vi "To Variant.vi"(0 "Base in":refnum<class "KDemoBase.lvclass">, 11 "error in (no error)":errorcluster) -> (4 "Base out":refnum<class "KDemoBase.lvclass">, 8 "Array":variant[](array[variant]), 15 "error out":errorcluster)   [LabVIEW 2015, in "KDemoBase.lvclass"]
uses:
  KDemoBase.lvclass
  KDemoBase.lvclass/KDemoBase.ctl
  KObject Class/KObject.lvclass
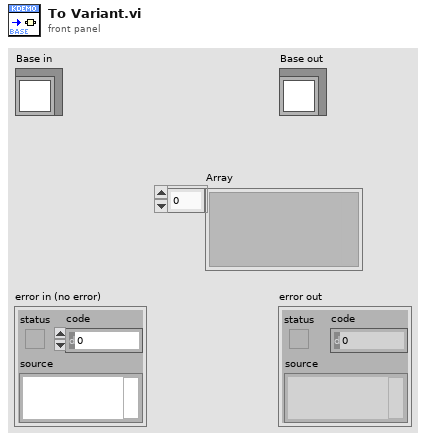
[diagram p1: front panel]
types:
  T1 = typedef "KDemoBase.lvclass/Serialized.ctl" = cluster{"Boolean":bool, "Value":dbl}
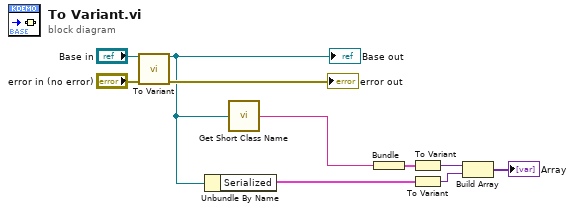
[diagram p0: block diagram]
diagram:
  n1 = call-parent "To Variant.vi"("KObject in"="Base in", "error in (no error)"="error in (no error)") -> ("KObject out"=w5:refnum<class "KDemoBase.lvclass">, "error out"=→"error out":errorcluster)  [unwired: 11 in, 1 out]
  "Base out" <- w5
  n2 = Unbundle By Name(w5) -> ("Serialized"=w3:T1)
  n3 = call "Get Short Class Name.vi"("KObject in"=w5) -> ("Class"=w2:string)  [unwired: 4 in]
  n4 = Bundle("Class"=w2) -> (w1:cluster{"Class":string})  [unwired: 1 in]
  n5 = To Variant(anything=w1) -> (Variant=w7:variant)
  n6 = To Variant(anything=w3) -> (Variant=w4:variant)
  n7 = Build Array(w7, w4) -> (→"Array":variant[])
